vi "pod_mode.vi"(11 "device ID":refnum<k1>) -> (0 "Curve":i32, 1 "Z":i32, 2 "speed":i32, 3 "command":string, 4 "ModeSelector  2":bool, 6 "P":bool, 7 "LegCluster":T1)   [LabVIEW 2014]
uses:
  <vilib>/Utility/inputDevices.llb/joystickAcquire.vi
panel:
  out "SingleLegTurn":i8
  out "SingleLegLift":i8
  out "SingleLegMode":bool=TRUE
  out "iteration 3":i32
  out "whichLeg":i32
  out "PWR":bool=TRUE
  out "iteration 2":i32
  out "PowerSelector":bool=TRUE
  out "iteration":i32
  out "ModeSelector":bool
  out "BasePosition":bool
  out "LegSelector":bool
  out "turbo":bool
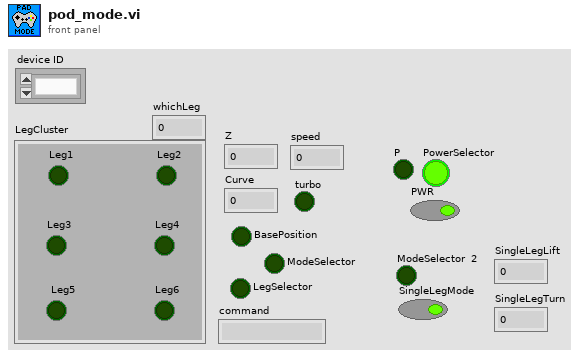
[diagram p1: front panel]
types:
  T1 = cluster{"Leg1":bool, "Leg2":bool, "Leg3":bool, "Leg4":bool, "Leg5":bool, "Leg6":bool}
  T2 = cluster{"X axis":i32, "Y axis":i32, "Z axis":i32, "X axis rotation":i32, "Y axis rotation":i32, "Z axis rotation":i32, "U axis":i32, "V axis":i32}
  T3 = cluster{"button 1":bool, "button 2":bool, "button 3":bool, "button 4":bool, "button 5":bool, "button 6":bool, "button 7":bool, "button 8":bool, "button 9":bool, "button 10":bool, "button 11":bool, "button 12":bool, "button 13":bool, "button 14":bool, "button 15":bool, "button 16":bool, "button 17":bool, "button 18":bool, "button 19":bool, "button 20":bool, "button 21":bool, "button 22":bool, "button 23":bool, "button 24":bool, "button 25":bool, "button 26":bool, "button 27":bool, "button 28":bool, "button 29":bool, "button 30":bool, "button 31":bool, "button 32":bool}
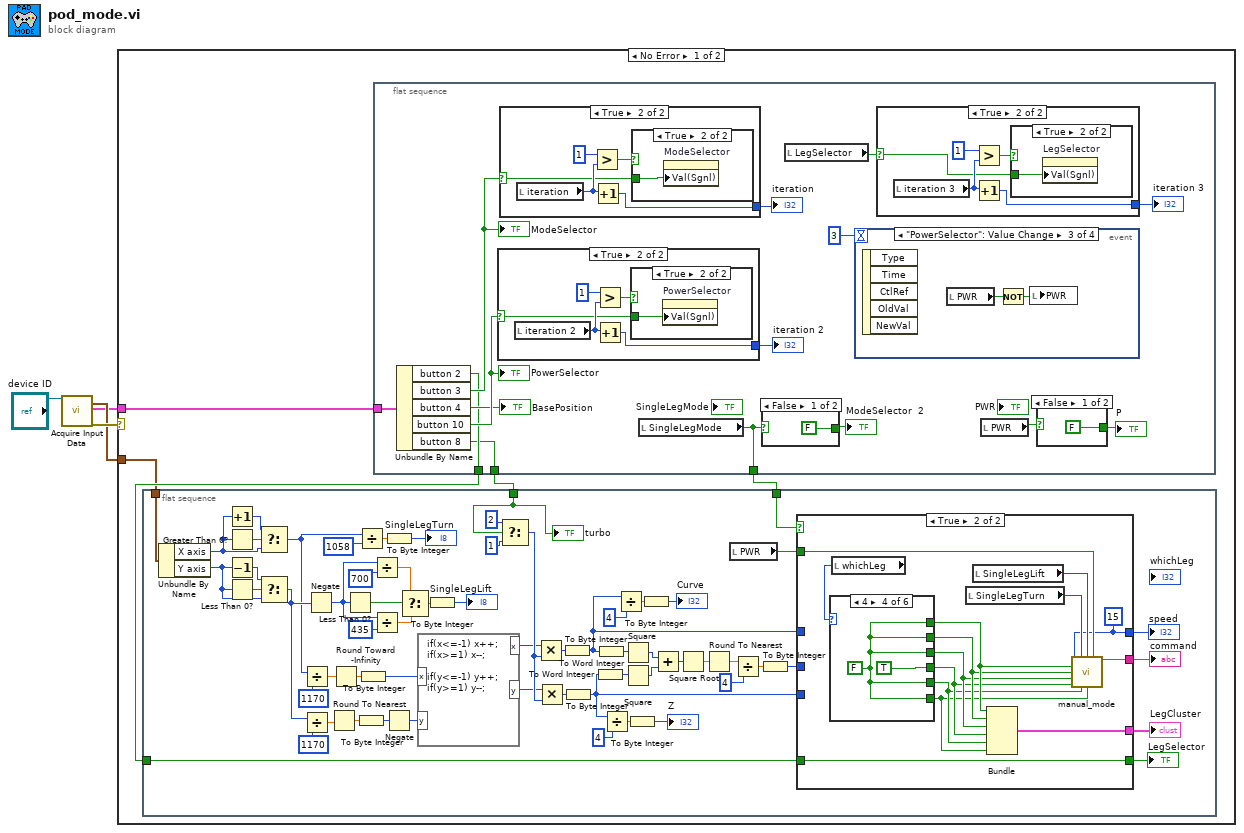
[diagram p0: block diagram]
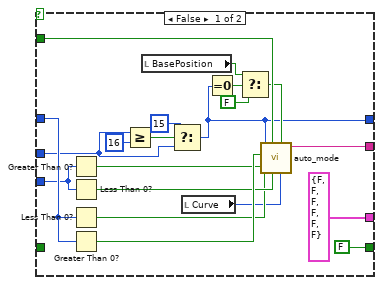
[diagram p2: hidden frame]
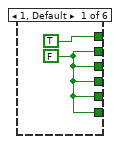
[diagram p3: hidden frame]
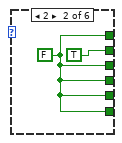
[diagram p4: hidden frame]
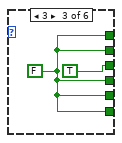
[diagram p5: hidden frame]
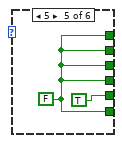
[diagram p6: hidden frame]
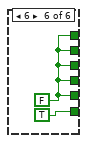
[diagram p7: hidden frame]
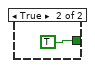
[diagram p8: hidden frame]
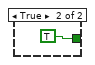
[diagram p9: hidden frame]
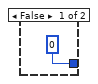
[diagram p10: hidden frame]
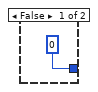
[diagram p12: hidden frame]
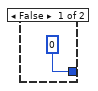
[diagram p14: hidden frame]
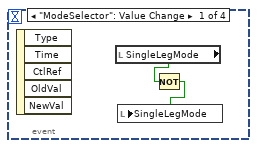
[diagram p16: hidden frame]
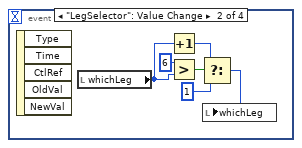
[diagram p17: hidden frame]
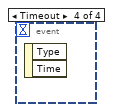
[diagram p18: hidden frame]
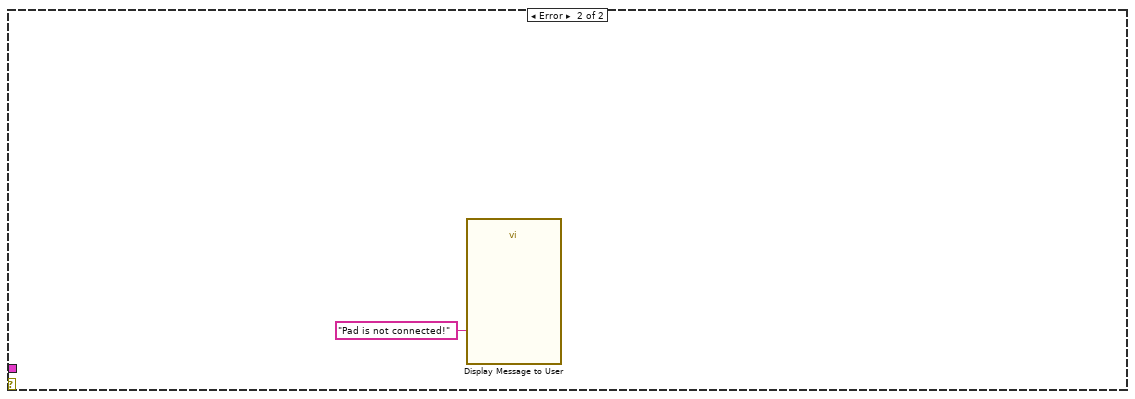
[diagram p19: hidden frame]
diagram:
  n1 = call-poly <vilib>:"Acquire Input Data.vi"("device ID"="device ID") -> ("axis info"=w2:T2, "button info"=w1:T3, "error out"=w3:errorcluster)  [unwired: 14 in, 2 out]
  n2 = case shown="No Error" w3 {
    tunnel: w2 -> [w6 _]
    tunnel: w1 -> [w5 _]
    frame No Error {
      n3 = flat-sequence {
        tunnel: w9 -> [w25]
        tunnel: w8 -> [w10]
        tunnel: w7 -> [w24]
        tunnel: w6 -> [w11]
        frame #0 {
          n4 = Unbundle By Name(w11) -> ("X axis"=w26:i32, "Y axis"=w27:i32)
          n5 = Increment(x=w26) -> (x+1=w35:i32)
          n6 = Greater Than 0?(x=w26) -> (x > 0?=w34:bool)
          n7 = Decrement(x=w27) -> (x-1=w33:i32)
          n8 = Less Than 0?(x=w27) -> (x < 0?=w32:bool)
          n9 = Select(t=w35, s=w34, f=w26) -> (s? t:f=w23:i32)
          n10 = Select(t=w33, s=w32, f=w27) -> (s? t:f=w70:i32)
          n11 = Divide(x=w23, y=1170) -> (x/y=w42:dbl)
          n12 = Divide(x=w70, y=1170) -> (x/y=w47:dbl)
          n13 = Negate(x=w70) -> (-x=w16:i32)
          n14 = Round To Nearest(number=w47) -> (nearest integer value=w46:dbl)
          n15 = Round Toward -Infinity(1:w42) -> (0:w43:dbl)
          n16 = Less Than 0?(x=w16) -> (x < 0?=w19:bool)
          n17 = To Byte Integer(number=w46) -> (8bit integer=w48:i8)
          n18 = Divide(x=w23, y=1058) -> (x/y=w21:dbl)
          n19 = To Byte Integer(number=w43) -> (8bit integer=w44:i8)
          n20 = Divide(x=w16, y=700) -> (x/y=w17:dbl)
          n21 = Divide(x=w16, y=435) -> (x/y=w14:dbl)
          n22 = To Byte Integer(number=w21) -> (8bit integer=→"SingleLegTurn":i8)
          n23 = Negate(x=w48) -> (-x=w40:i8)
          n24 = Select(t=w17, s=w19, f=w14) -> (s? t:f=w13:dbl)
          n25 = formula code="if(x<=-1) x++;\nif(x>=1) x--;\n\nif(y<=-1) y++;\nif(y>=1) y--;"("x"=w44, "y"=w40) -> ("x"=w49:i8, "y"=w39:i8)
          n26 = To Byte Integer(number=w13) -> (8bit integer=→"SingleLegLift":i8)
          n27 = Select(t=u8 2, s=w10, f=u8 1) -> (s? t:f=w50:u8)
          n28 = Multiply(x=w49, y=w50) -> (x*y=w51:u8)
          n29 = Multiply(x=w39, y=w50) -> (x*y=w52:u8)
          n30 = To Byte Integer(number=w51) -> (8bit integer=w68:i8)
          n31 = To Byte Integer(number=w52) -> (8bit integer=w67:i8)
          n32 = To Word Integer(number=w67) -> (16bit integer=w63:i16)
          n33 = To Word Integer(number=w68) -> (16bit integer=w62:i16)
          n34 = Divide(x=w67, y=u8 4) -> (x/y=w56:dbl)
          n35 = Divide(x=w68, y=u8 4) -> (x/y=w54:dbl)
          n36 = Square(x=w62) -> (x^2=w60:i16)
          n37 = Square(x=w63) -> (x^2=w61:i16)
          n38 = To Byte Integer(number=w56) -> (8bit integer=→"Z":i8)
          n39 = To Byte Integer(number=w54) -> (8bit integer=→"Curve":i8)
          n40 = Add(x=w60, y=w61) -> (x+y=w59:i16)
          n41 = Square Root(x=w59) -> (sqrt(x)=w58:dbl)
          n42 = Round To Nearest(number=w58) -> (nearest integer value=w65:dbl)
          n43 = local read "PWR"() -> (w29:bool)
          n44 = Divide(x=w65, y=u8 4) -> (x/y=w66:dbl)
          n45 = To Byte Integer(number=w66) -> (8bit integer=w69:i8)
          n46 = case shown="True" w24 {
            tunnel: [FALSE ("button 2") w103] -> w28
            tunnel: w29 -> [w90 w105]
            tunnel: [w89 w104] -> w30
            tunnel: [w72 w92] -> w31
            tunnel: w67 -> [w78 _]
            tunnel: w68 -> [w79 _]
            tunnel: w25 -> [_ w103]
            tunnel: [cluster{bool, bool, bool, bool, bool, bool} {FALSE, FALSE, FALSE, FALSE, FALSE, FALSE} w95] -> w38
            tunnel: w69 -> [w73 _]
            frame False {
              n47 = Greater Than 0?(x=w78) -> (x > 0?=w86:bool)
              n48 = Less Than 0?(x=w78) -> (x < 0?=w87:bool)
              n49 = Less Than 0?(x=w79) -> (x < 0?=w80:bool)
              n50 = Greater Than 0?(x=w79) -> (x > 0?=w88:bool)
              n51 = Greater Or Equal?(x=w73, y=i8 16) -> (x >= y?=w76:bool)
              n52 = local read "BasePosition"() -> (w84:bool)
              n53 = Select(t=i8 15, s=w76, f=w73) -> (s? t:f=w72:i8)
              n54 = local read "Curve"() -> (w77:i32)
              n55 = Equal To 0?(x=w72) -> (x = 0?=w82:bool)
              n56 = Select(t=w84, s=w82, f=FALSE) -> (s? t:f=w85:bool)
              n57 = call "auto_mode.vi"("Curve"=w77, "Base Position"=w85, "Back"=w87, "POWER"=w90, "Right"=w80, "Forth"=w86, "Left"=w88, "Speed"=w72) -> ("String"=w89:string)  [unwired: 3 in]
            }
            frame True {
              w92 = u8 15 ("Speed")
              n58 = local read "whichLeg"() -> (w102:i32)
              n59 = case shown="4" w102 {
                tunnel: [TRUE w108 w110 w112 w114 w116] -> w101
                tunnel: [w106 TRUE w110 w112 w114 w116] -> w100
                tunnel: [w106 w108 TRUE w112 w114 w116] -> w99
                tunnel: [w106 w108 w110 TRUE w114 w116] -> w98
                tunnel: [w106 w108 w110 w112 TRUE w116] -> w97
                tunnel: [w106 w108 w110 w112 w114 TRUE] -> w96
                frame 1, Default {
                  w106 = FALSE
                }
                frame 2 {
                  w108 = FALSE
                }
                frame 3 {
                  w110 = FALSE
                }
                frame 4 {
                  w112 = FALSE
                }
                frame 5 {
                  w114 = FALSE
                }
                frame 6 {
                  w116 = FALSE
                }
              }
              n60 = local read "SingleLegTurn"() -> (w94:i8)
              n61 = local read "SingleLegLift"() -> (w93:i8)
              n62 = Bundle(w101, w100, w99, w98, w97, w96) -> (w95:cluster{bool, bool, bool, bool, bool, bool})  [unwired: 1 in]
              n63 = call "manual_mode.vi"("Speed"=w92, "Turn"=w94, "Lift"=w93, "POWER"=w105, "LEG1"=w101, "LEG2"=w100, "LEG3"=w99, "LEG4"=w98, "LEG5"=w97, "LEG6"=w96) -> ("String"=w104:string)  [unwired: 5 in]
            }
          }
          "LegSelector" <- w28
          "command" <- w30
          "speed" <- w31
          "LegCluster" <- w38
          "turbo" <- w10
        }
      }
      n64 = flat-sequence {
        tunnel: [w124] -> w9
        tunnel: [w123] -> w7
        tunnel: [w122] -> w8
        tunnel: w5 -> [w121]
        frame #0 {
          n65 = Unbundle By Name(w121) -> ("button 2"=w124:bool, "button 3"=w130:bool, "button 4"=→"BasePosition":bool, "button 10"=w131:bool, "button 8"=w122:bool)
          "ModeSelector" <- w130
          "PowerSelector" <- w131
          n66 = case shown="True" w131 {
            selector: w131 -> [_ w146]
            tunnel: [0 ("iteration") w145] -> w118
            frame False {
            }
            frame True {
              n67 = local read "iteration 2"() -> (w147:i32)
              n68 = Greater?(x=u32 1, y=w147) -> (0:w149:bool)
              n69 = Increment(x=w147) -> (x+1=w145:i32)
              n70 = case shown="True" w149 {
                tunnel: w146 -> [_ w150]
                frame False {
                }
                frame True {
                  n71 = property on="PowerSelector" class="Bool (strict)"("Val(Sgnl)"=w150) -> ()  [unwired: 2 in, 2 out]
                }
              }
            }
          }
          "iteration 2" <- w118
          n72 = case shown="True" w130 {
            selector: w130 -> [_ w153]
            tunnel: [0 ("iteration") w152] -> w119
            frame False {
            }
            frame True {
              n73 = local read "iteration"() -> (w154:i32)
              n74 = Greater?(x=u32 1, y=w154) -> (0:w156:bool)
              n75 = Increment(x=w154) -> (x+1=w152:i32)
              n76 = case shown="True" w156 {
                tunnel: w153 -> [_ w157]
                frame False {
                }
                frame True {
                  n77 = property on="ModeSelector" class="Bool (strict)"("Val(Sgnl)"=w157) -> ()  [unwired: 2 in, 2 out]
                }
              }
            }
          }
          "iteration" <- w119
          n78 = local read "SingleLegMode"() -> (w123:bool)
          n79 = case shown="False" w123 {
            tunnel: [FALSE TRUE] -> w127
            frame False {
            }
            frame True {
            }
          }
          "ModeSelector  2" <- w127
          n80 = local read "LegSelector"() -> (w132:bool)
          n81 = event shown="[2] \"PowerSelector\": Value Change" {
            selector: _ -> [_ _ _ _]
            dyn-events: _ -> [_ _ _ _]
            timeout: 3 -> [_ _ _ _]
            event "ModeSelector": Value Change {
              n82 = event-data() -> ()  [unwired: 1 in, 5 out]
              n83 = local read "SingleLegMode"() -> (w158:bool)
              n84 = Not(x=w158) -> (.not. x?=w159:bool)
              n85 = local write "SingleLegMode"(w159) -> ()
            }
            event "LegSelector": Value Change {
              n86 = event-data() -> ()  [unwired: 1 in, 5 out]
              n87 = local read "whichLeg"() -> (w163:i32)
              n88 = Increment(x=w163) -> (x+1=w162:i32)
              n89 = Greater?(x=6 ("y"), y=w163) -> (0:w165:bool)
              n90 = Select(t=w162, s=w165, f=1) -> (s? t:f=w160:i32)
              n91 = local write "whichLeg"(w160) -> ()
            }
            event "PowerSelector": Value Change {
              n92 = event-data() -> ()  [unwired: 1 in, 5 out]
              n93 = local read "PWR"() -> (w167:bool)
              n94 = Not(x=w167) -> (.not. x?=w166:bool)
              n95 = local write "PWR"(w166) -> ()
            }
            event Timeout {
              n96 = event-data() -> ()  [unwired: 1 in, 2 out]
            }
          }
          n97 = case shown="True" w132 {
            selector: w132 -> [_ w139]
            tunnel: [0 ("iteration") w138] -> w120
            frame False {
            }
            frame True {
              n98 = local read "iteration 3"() -> (w140:i32)
              n99 = Greater?(x=u32 1, y=w140) -> (0:w142:bool)
              n100 = Increment(x=w140) -> (x+1=w138:i32)
              n101 = case shown="True" w142 {
                tunnel: w139 -> [_ w143]
                frame False {
                }
                frame True {
                  n102 = property on="LegSelector" class="Bool (strict)"("Val(Sgnl)"=w143) -> ()  [unwired: 2 in, 2 out]
                }
              }
            }
          }
          "iteration 3" <- w120
          n103 = local read "PWR"() -> (w126:bool)
          n104 = case shown="False" w126 {
            tunnel: [FALSE TRUE] -> w125
            frame False {
            }
            frame True {
            }
          }
          "P" <- w125
        }
      }
    }
    frame Error {
      n105 = call "Display Message to User"("Message"="Pad is not connected!") -> ()  [unwired: 9 in, 2 out]
    }
  }
